vi "Write config_DVR.vi"(8 "error in (no error)":errorcluster, 10 "config_DVR":refnum<data-value>, 11 "PredictiveMaintenance.lvlib:PredictiveMaintenance.lvclass":refnum<class "PredictiveMaintenance.lvclass">) -> (0 "error out":errorcluster, 3 "PredictiveMaintenance.lvlib:PredictiveMaintenance.lvclass 2":refnum<class "PredictiveMaintenance.lvclass">)   [LabVIEW 2019, in "PredictiveMaintenance.lvlib" / "PredictiveMaintenance.lvclass"]
uses:
  PredictiveMaintenance.lvclass
  ConfigClass/ConfigClass/ConfigClass.lvclass
  PredictiveMaintenance.lvclass/PredictiveMaintenance.ctl
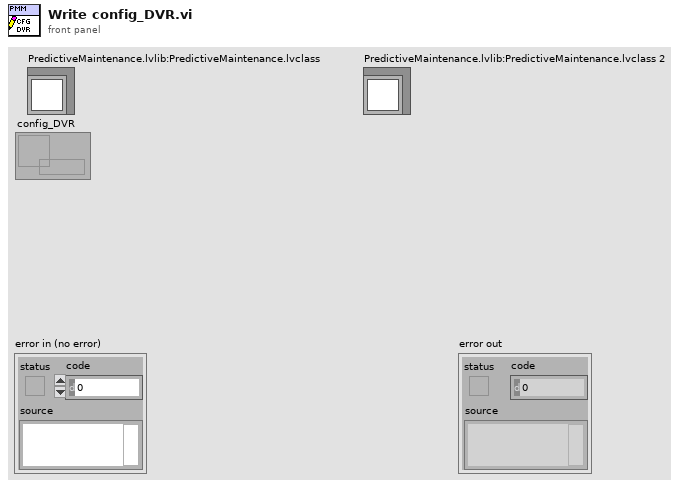
[diagram p1: front panel]
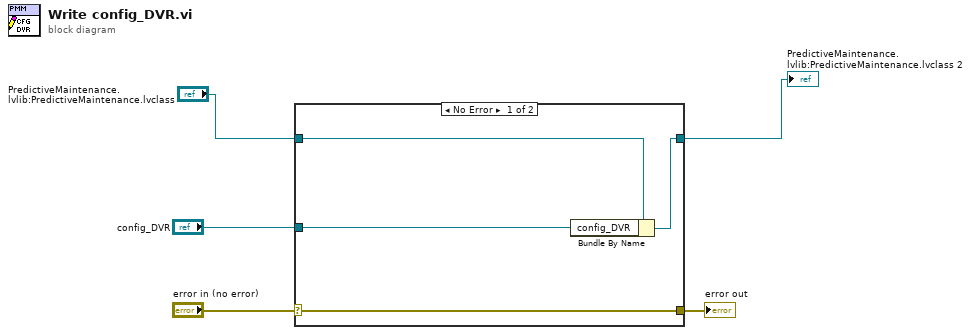
[diagram p0: block diagram]
diagram:
  n1 = case shown="No Error" "error in (no error)" {
    selector: "error in (no error)" -> [w9 w10]
    tunnel: [w9 w10] -> w4
    tunnel: [w7 w11] -> w1
    tunnel: "PredictiveMaintenance.lvlib:PredictiveMaintenance.lvclass" -> [w8 w11]
    tunnel: "config_DVR" -> [w6 _]
    frame No Error {
      n2 = Bundle By Name(cluster=w8, "config_DVR"=w6) -> (w7:refnum<class "PredictiveMaintenance.lvclass">)
    }
    frame Error {
    }
  }
  "error out" <- w4
  "PredictiveMaintenance.lvlib:PredictiveMaintenance.lvclass 2" <- w1
